vi "Write encoderCounts.vi"(10 "encoderCounts":i32, 11 "EnccoderConverter in":refnum<class "EncoderConverter.lvclass">) -> (3 "EnccoderConverter out":refnum<class "EncoderConverter.lvclass">)   [LabVIEW 2013, in "EncoderConverter.lvlib" / "EncoderConverter.lvclass"]
uses:
  <userlib>/Common/Devices/EncoderConverter/EncoderConverter/EncoderConverter.lvclass
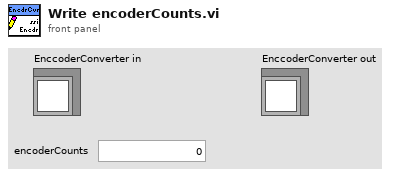
[diagram p1: front panel]
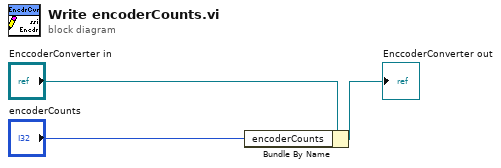
[diagram p0: block diagram]
diagram:
  n1 = Bundle By Name(cluster="EnccoderConverter in", "encoderCounts"="encoderCounts") -> (→"EnccoderConverter out":refnum<class "EncoderConverter.lvclass">)
